vi "Subvi stage distance trigger.vi"(8 "StageMotionMonitor":bool, 10 "StagePositionMonitor":bool) -> (2 "Trigger":bool)   [LabVIEW 2017]
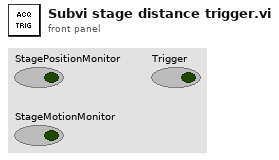
[diagram p1: front panel]
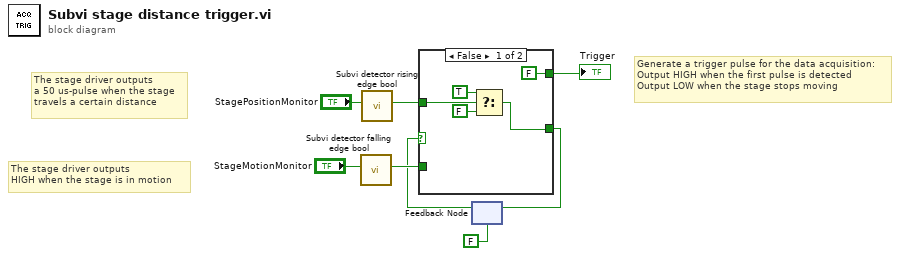
[diagram p0: block diagram]
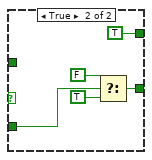
[diagram p2: hidden frame]
diagram:
  # "The stage driver outputs\na 50 us-pulse when the stage\ntravels a certain distance"
  # "The stage driver outputs\nHIGH when the stage is in motion"
  # "Generate a trigger pulse for the data acquisition:\nOutput HIGH when the first pulse is detected\nOutput LOW when the stage stops moving"
  n1 = call "Subvi detector falling edge bool.vi"("Input"="StageMotionMonitor") -> ("Output"=w7:bool)  [unwired: 10 in]
  n2 = call "Subvi detector rising edge bool.vi"("Input"="StagePositionMonitor") -> ("Output"=w5:bool)  [unwired: 10 in]
  n3 = feedback #1(FALSE) -> (w6:bool)
  n4 = case shown="False" w6 {
    tunnel: [w12 w17] -> w4
    tunnel: w5 -> [w13 _]
    tunnel: w7 -> [_ w18]
    tunnel: [FALSE TRUE] -> w8
    frame False {
      n5 = Select(t=TRUE, s=w13, f=FALSE) -> (s? t:f=w12:bool)
    }
    frame True {
      n6 = Select(t=FALSE, s=w18, f=TRUE) -> (s? t:f=w17:bool)
    }
  }
  "Trigger" <- w8
  n7 = feedback-in #1(w4) -> ()
